vi "SetCameraAQ.vi"(8 "error in":errorcluster, 11 "Camera":T1={"Gate.Delay"=0, "Delay.Step"=0, "Gate.Duration"=150000, "#Accum"=10, "SetpointTemp"=-30, "Last Temp"=6, "Current Temp"=4}) -> (0 "error out":errorcluster, 3 "Camera out":T1={"Gate.Delay"=0, "Delay.Step"=0, "Gate.Duration"=150000, "#Accum"=10, "SetpointTemp"=-30, "Last Temp"=6, "Current Temp"=4})   [LabVIEW 2022 SP3]
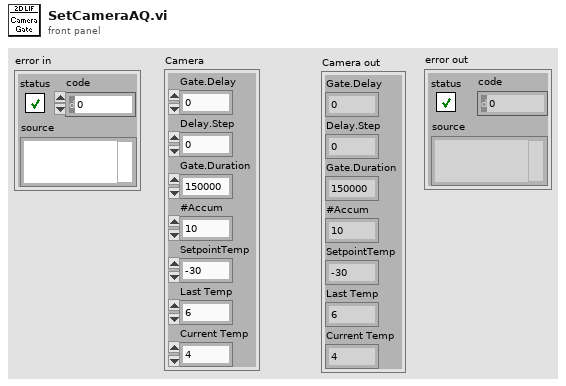
[diagram p1: front panel]
types:
  T1 = cluster{"Gate.Delay":u64, "Delay.Step":u64, "Gate.Duration":u64, "#Accum":i32, "SetpointTemp":i32, "Last Temp":i32, "Current Temp":i32}
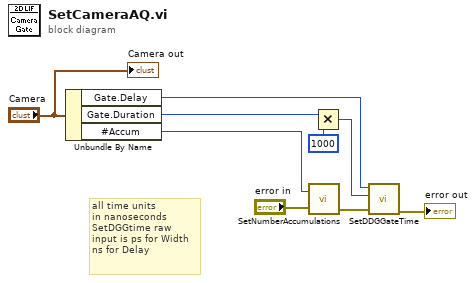
[diagram p0: block diagram]
diagram:
  # "all time units\nin nanoseconds\nSetDGGtime raw\ninput is ps for Width\nns for Delay"
  n1 = Unbundle By Name("Camera") -> ("Gate.Delay"=w7:u64, "Gate.Duration"=w4:u64, "#Accum"=w6:i32)
  n2 = call "SetNumberAccumulations.vi"("error in (no error)"="error in", "number"=w6) -> ("error out"=w9:errorcluster)  [unwired: 1 out]
  n3 = Multiply(x=w4, y=u64 1000) -> (x*y=w3:u64)
  n4 = call "SetDDGGateTime.vi"("error in (no error)"=w9, "Width"=w3, "Delay"=w7) -> ("error out"=→"error out":errorcluster)  [unwired: 7 in, 1 out]
  "Camera out" <- "Camera"
